vi "MC Cycle Engine Request State ERD.vi"(0 "GEA2 Reference In":refnum<k24>, 1 "GEA Inputs":T2 {"Destination" format="%.0x"; "Source" format="%.0x"}, 2 "Standalone?":bool, 7 "Cycle #":u8, 9 "MC Cycle Engine State":T1, 11 "Error In":errorcluster) -> (4 "GEA2 Reference Out":refnum<k24>, 15 "Error Out":errorcluster)   [LabVIEW 2016, in "Centauro.lvlib"]
doc: "This vi can be used to update the MC cycle engine state with the requested values."
uses:
  Projects/Centauro.lvlib
  Q:/Common/DLLs/GEA3/GeaCommunication.dll
  Common/DLLs/GEA3/GeaCommunication.dll
  Common/LabVIEW GEA2 Toolkit/LabVIEW_GEA2_Toolkit.lvlibp/type defs/Source_Destination.ctl
  type defs/MC_Cycle_Engine_Request_State.ctl
  Common/LabVIEW GEA2 Toolkit/LabVIEW_GEA2_Toolkit.lvlibp/type defs/ERD Write Data In.ctl
  Common/LabVIEW GEA2 Toolkit/LabVIEW_GEA2_Toolkit.lvlibp/type defs/Data Type.ctl
  Common/LabVIEW GEA2 Toolkit/LabVIEW_GEA2_Toolkit.lvlibp
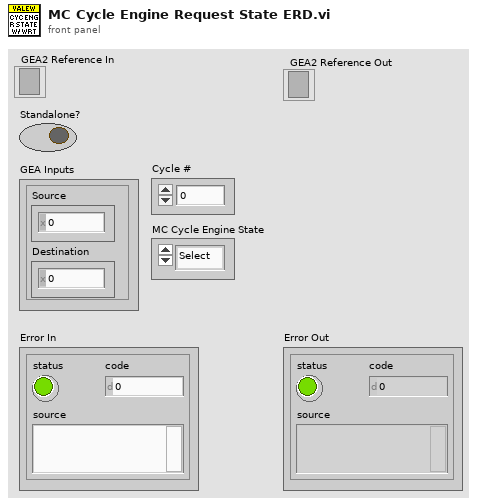
[diagram p1: front panel]
types:
  T1 = typedef "Centauro.lvlib/MC_Cycle_Engine_Request_State.ctl" = enum16{"Select", "Start", "Pause", "Resume", "Stop"}
  T2 = typedef "LabVIEW_GEA2_Toolkit.lvlibp/Source_Destination.ctl" = cluster{"Source":u8, "Destination":u8}
  T3 = typedef "LabVIEW_GEA2_Toolkit.lvlibp/ERD Write Data In.ctl" = cluster{"ERD Number":u16, "Data Type":T4, "Data":string}
  T4 = typedef "LabVIEW_GEA2_Toolkit.lvlibp/Data Type.ctl" = enum16{"string", "boolean", "uint8_t", "uint16_t", "uint32_t", "uint64_t", "int8_t", "int16_t", "int32_t", "int64_t"}
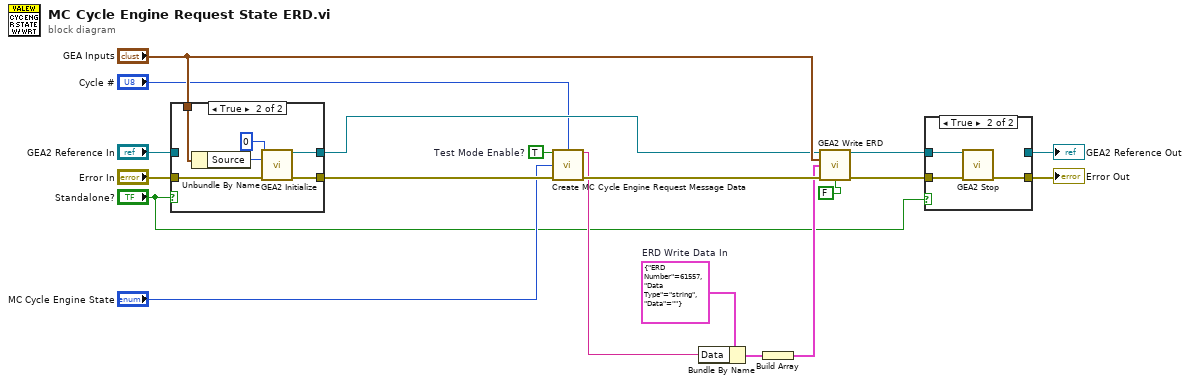
[diagram p0: block diagram]
diagram:
  w2 = TRUE  # Test Mode Enable?
  w18 = T3 {"ERD Number"=61557, "Data Type"=enum."string", "Data"=""}  # ERD Write Data In
  n1 = case shown="True" "Standalone?" {
    tunnel: "Error In" -> [w20 w27]
    tunnel: [w20 w26] -> w15
    tunnel: "GEA2 Reference In" -> [w21 _]
    tunnel: [w21 w25] -> w13
    tunnel: "GEA Inputs" -> [_ w23]
    frame False {
    }
    frame True {
      n2 = Unbundle By Name(w23) -> ("Source"=w24:u8)
      n3 = call "GEA2 Initialize.vi"("Board Index"=0, "Source Address"=w24, "error in"=w27) -> ("GEA2 Reference Out"=w25:refnum<k24>, "error out"=w26:errorcluster)  [unwired: 10 in, 1 out]
    }
  }
  n4 = call "Create MC Cycle Engine Request Message Data .vi"("Test Mode Enable?"=w2, "Cycle #"="Cycle #", "MC Cycle Engine State"="MC Cycle Engine State", "Error In"=w15) -> ("MC Cycle Engine Request Message Data"=w12:string, "Error Out"=w14:errorcluster)  [unwired: 10 in]
  n5 = Bundle By Name(cluster=w18, "Data"=w12) -> (w8:T3)
  n6 = Build Array(w8) -> (w9:T3[])
  n7 = call "GEA2 Write ERD.vi"("GEA2 Reference In"=w13, "GEA Inputs"="GEA Inputs", "Write ERD List"=w9, "Error In"=w14, "Verify ERD Response?"=FALSE) -> ("GEA2 Reference Out"=w16:refnum<k24>, "Error Out"=w17:errorcluster)  [unwired: 8 in, 1 out]
  n8 = case shown="True" "Standalone?" {
    tunnel: w17 -> [w28 w32]
    tunnel: [w28 w31] -> w7
    tunnel: w16 -> [w29 w30]
    tunnel: [w29 _] -> w6
    frame False {
    }
    frame True {
      n9 = call "GEA2 Stop.vi"("GEA2 Reference In"=w30, "Error In"=w32) -> ("Error Out"=w31:errorcluster)  [unwired: 13 in]
    }
  }
  "Error Out" <- w7
  "GEA2 Reference Out" <- w6
